vi "Mono Slit.vi"(8 "error in (no error)":errorcluster, 11 "Mono In":refnum<class "Monochromator.lvclass">) -> (0 "error out":errorcluster, 2 "new position":dbl, 3 "position":dbl)   [LabVIEW 2020, in "Examples.lvlib"]
doc: "This example shows how to get and set the slit width of the mono."
uses:
  Examples.lvlib
  Classes/Mono/Monochromator.lvclass
  1e589c04-ee94-437c-90d0-11a3ef27d9f2.vi
  98d9e02b-2768-4993-9cff-527122a95b91.vi
panel:
  in  "Stop":bool
  # "Connector Pane"
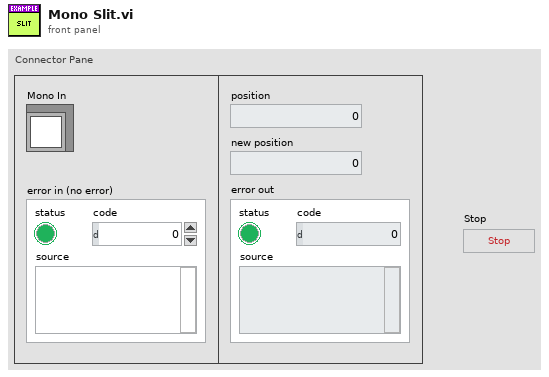
[diagram p1: front panel]
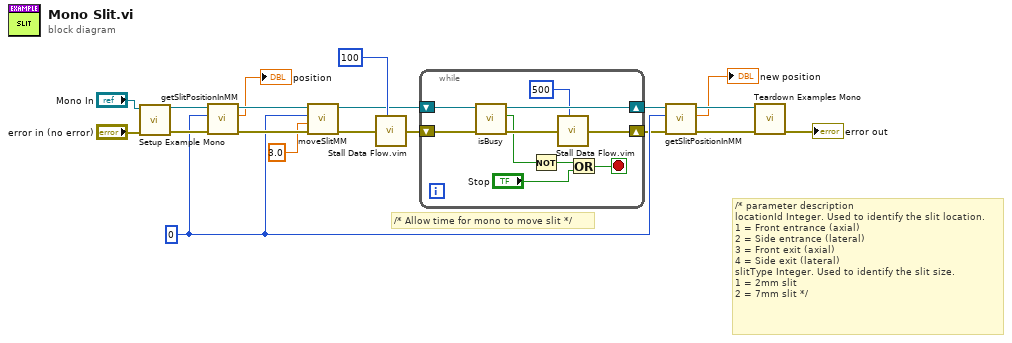
[diagram p0: block diagram]
diagram:
  w7 = 0 ("locationId")
  # "/* parameter\tdescription\nlocationId\tInteger. Used to identify the slit location.\n1 = Front entrance (axial)\n2 = Side entrance (lateral)\n3 = Front exit (axial)\n4 = Side exit (lateral)\nslitType\tInteger. Used to identify the slit size.\n1 = 2mm slit\n2 = 7mm slit */"
  # "/* Allow time for mono to move slit */"
  n1 = call "Setup Example Mono.vi"("error in (no error)"="error in (no error)", "Mono In"="Mono In") -> ("error out"=w16:errorcluster, "Mono Out"=w14:refnum<class "Monochromator.lvclass">)  [unwired: 6 in, 2 out]
  n2 = call "getSlitPositionInMM.vi"("error in (no error)"=w16, "locationId"=w7, "Monochromator in"=w14) -> ("error out"=w15:errorcluster, "position"=→"position":dbl, "Monochromator out"=w13:refnum<class "Monochromator.lvclass">)  [unwired: 6 in]
  n3 = call "moveSlitMM.vi"("error in (no error)"=w15, "position"=3.0, "locationId"=w7, "Monochromator in"=w13) -> ("error out"=w12:errorcluster, "Monochromator out"=w3:refnum<class "Monochromator.lvclass">)  [unwired: 4 in, 2 out]
  n4 = call "Stall Data Flow.vim"("value in"=w12, "milliseconds to wait"=u32 100) -> ("value out"=w4:errorcluster)  [unwired: 1 out]
  n5 = while {
    shift-right: [w25] -> w1
    shift-left: w4 -> [w27]
    shift-right: [w28] -> w2
    shift-left: w3 -> [w26]
    stop <- w22 stop-if-true
    n6 = call "isBusy.vi"("error in (no error)"=w27, "Monochromator in"=w26) -> ("error out"=w29:errorcluster, "mono is busy?"=w23:bool, "Monochromator out"=w28:refnum<class "Monochromator.lvclass">)  [unwired: 7 in]
    n7 = Not(x=w23) -> (.not. x?=w20:bool)
    n8 = call "Stall Data Flow.vim"("value in"=w29, "milliseconds to wait"=u32 500) -> ("value out"=w25:errorcluster)  [unwired: 1 out]
    n9 = Or(x=w20, y="Stop") -> (x .or. y?=w22:bool)
  }
  n10 = call "getSlitPositionInMM.vi"("error in (no error)"=w1, "locationId"=w7, "Monochromator in"=w2) -> ("error out"=w9:errorcluster, "position"=→"new position":dbl, "Monochromator out"=w8:refnum<class "Monochromator.lvclass">)  [unwired: 6 in]
  n11 = call "Teardown Examples Mono.vi"("error in (no error)"=w9, "Monochromator in"=w8) -> ("error out"=→"error out":errorcluster)  [unwired: 9 in]
